vi "Last Target String.vi"(8 "error in (no error)":errorcluster, 11 "TargetPluginManager in":refnum<class "PlatformPluginManager.lvclass">) -> (0 "error out":errorcluster, 2 "Last Target String":string, 3 "TargetPluginManager out":refnum<class "PlatformPluginManager.lvclass">)   [LabVIEW 2020, in "PicoG-Core.lvlib" / "PlatformPluginManager.lvclass"]
uses:
  PlatformPluginManager.lvclass
  PlatformPluginManager.lvclass/PlatformPluginManager.ctl
  DeployPlatform/DeployPlatform.lvclass
  DeployResource/DeployResource.lvclass
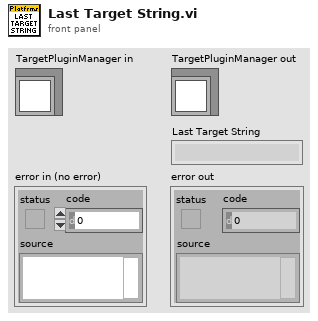
[diagram p1: front panel]
types:
  T1 = typedef "PicoG-Core.lvlib/PlatformPluginManager.lvclass/Ref Data.ctl" = cluster{"Platforms":refnum<class "DeployPlatform.lvclass">[], "Last Platform":refnum<class "DeployPlatform.lvclass">, "Last Resource":refnum<class "DeployResource.lvclass">}
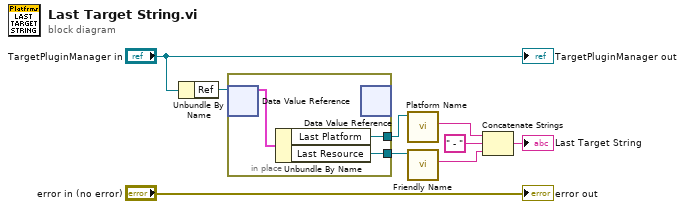
[diagram p0: block diagram]
diagram:
  n1 = Unbundle By Name("TargetPluginManager in") -> ("Ref"=w8:refnum<data-value>)
  n2 = in-place {
    in-place-border: [w11] -> w6
    in-place-border: [w10] -> w5
    n3 = in-place-dvr #1(w8) -> (w12:T1)  [unwired: 1 out]
    n4 = Unbundle By Name(w12) -> ("Last Platform"=w11:refnum<class "DeployPlatform.lvclass">, "Last Resource"=w10:refnum<class "DeployResource.lvclass">)
    n5 = in-place-dvr #1() -> ()  [unwired: 1 in, 2 out]
  }
  n6 = call-dynamic "Platform Name.vi"("DeployTarget in"=w6) -> ("Platform Name"=w3:string)  [unwired: 8 in, 2 out]
  n7 = call-dynamic "Friendly Name.vi"("DeployResource in"=w5) -> ("Friendly Name"=w2:string)  [unwired: 8 in, 2 out]
  n8 = Concatenate Strings(w3, " - " ("string"), w2) -> (→"Last Target String":string)
  "error out" <- "error in (no error)"
  "TargetPluginManager out" <- "TargetPluginManager in"
